vi "Open.vi"(8 "error in (no error)":errorcluster, 11 "VISA resource name":refnum<visa-resource-name>) -> (0 "error out":errorcluster, 3 "VISA resource":refnum<visa-resource-name>)   [LabVIEW 2019, in "KH7008.lvlib"]
uses:
  KH7008.lvlib
  <vilib>/Instr/_visa.llb/VISA Configure Serial Port (Instr).vi
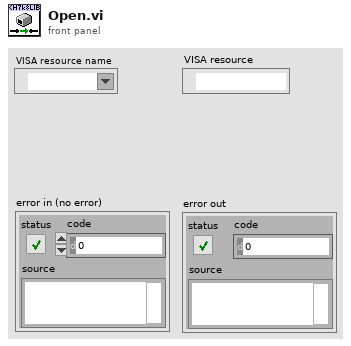
[diagram p1: front panel]
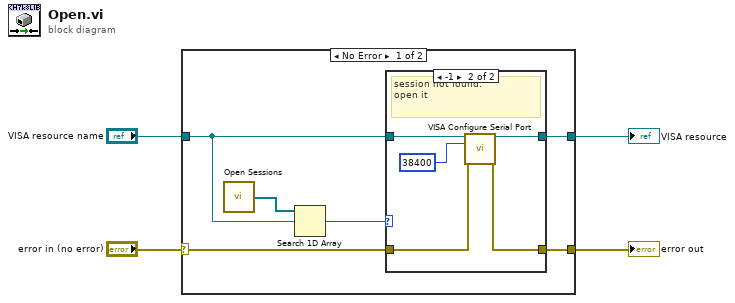
[diagram p0: block diagram]
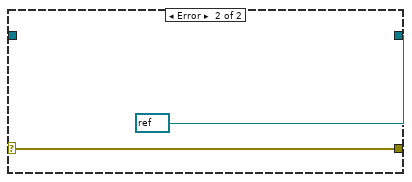
[diagram p3: hidden frame]
diagram:
  n1 = case shown="No Error" "error in (no error)" {
    selector: "error in (no error)" -> [w7 w19]
    tunnel: [w10 refnum<visa-resource-name> refnum ("VISA resource name out")] -> w4
    tunnel: [w9 w19] -> w3
    tunnel: "VISA resource name" -> [w6 _]
    frame No Error {
      n2 = call <vilib>:"Open Sessions.vi"() -> ("Array of Refnums"=w8:refnum<visa-resource-name>[])  [unwired: 2 in]
      n3 = Search 1D Array(1D array=w8, element=w6) -> (index of element=w5:i32)  [unwired: 1 in]
      n4 = case shown="-1" w5 {
        tunnel: [w12 w16] -> w10
        tunnel: [w11 w15] -> w9
        tunnel: w7 -> [w11 w14]
        tunnel: w6 -> [w12 w13]
        frame 0, Default {
          # "session found:\ndo not open again"
        }
        frame -1 {
          # "session not found:\nopen it"
          n5 = call-poly "VISA Configure Serial Port"("VISA resource name"=w13, "baud rate (9600)"=u32 38400, "error in (no error)"=w14) -> ("VISA resource name out"=w16:refnum<visa-resource-name>, "error out"=w15:errorcluster)  [unwired: 6 in, 5 out]
        }
      }
    }
    frame Error {
    }
  }
  "VISA resource" <- w4
  "error out" <- w3
